vi "Configure Digital Audio Reference.vi"(8 "error in (no error)":errorcluster, 9 "User Input Sampling Rate Ref (0 kHz)":i32, 10 "Input Sampling Rate Ref (0: dioGenerator)":i32(ring) items=["dioGenerator", "dioMeasured", "dioStatusBits", "dioUser"], 11 "VISA resource name":refnum<visa-resource-name>) -> (0 "error out":errorcluster, 3 "VISA resource name out":refnum<visa-resource-name>)   [LabVIEW 2014, in "Stanford Research SR1.lvlib"]
doc: "Configures the sampling reference settings for Digital Audio."
uses:
  Stanford Research SR1.lvlib
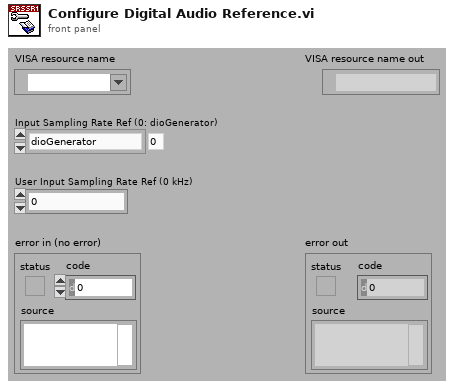
[diagram p1: front panel]
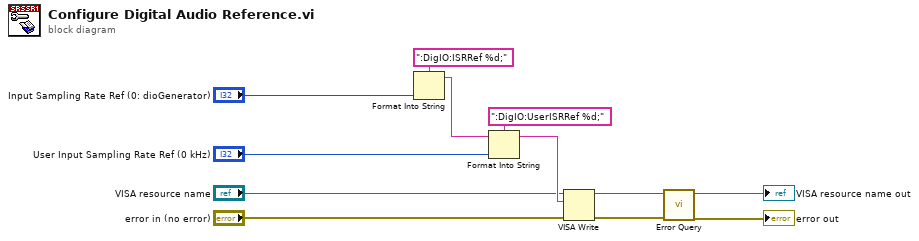
[diagram p0: block diagram]
diagram:
  n1 = Format Into String(format string=":DigIO:ISRRef %d;", "Input Sampling Rate Ref (0: dioGenerator)") -> (resulting string=w10:string)  [unwired: 2 in, 1 out]
  n2 = Format Into String(format string=":DigIO:UserISRRef %d;", initial string=w10, "User Input Sampling Rate Ref (0 kHz)") -> (resulting string=w7:string)  [unwired: 1 in, 1 out]
  n3 = VISA Write(VISA resource name="VISA resource name", write buffer=w7, error in (no error)="error in (no error)") -> (VISA resource name out=w4:refnum<visa-resource-name>, error out=w3:errorcluster)  [unwired: 1 out]
  n4 = call "Error Query.vi"("error in (no error)"=w3, "VISA resource name"=w4) -> ("error out"=→"error out":errorcluster, "VISA resource name out"=→"VISA resource name out":refnum<visa-resource-name>)  [unwired: 6 in, 2 out]
